vi "Flow_velocity_write.vi"(3 "error in":errorcluster) -> (0 "error out":errorcluster)   [LabVIEW 2013]
uses:
  <vilib>/Analysis/NI_AALPro.lvlib
  <vilib>/Analysis/_algsub.llb/Real Vector Norm.vi
panel:
  in  "NSensors":i32
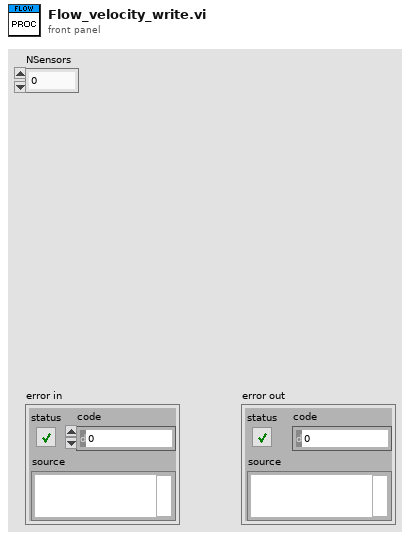
[diagram p1: front panel]
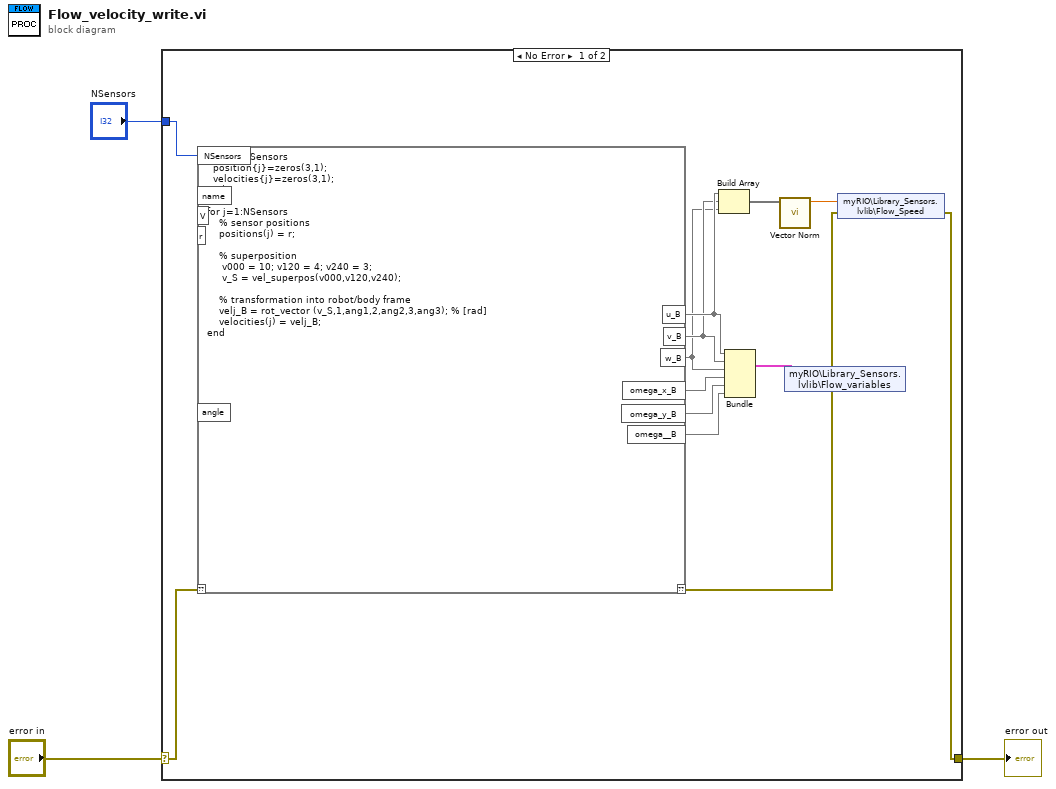
[diagram p0: block diagram]
diagram:
  n1 = case shown="No Error" "error in" {
    selector: "error in" -> [w6 w17]
    tunnel: [w4 w17] -> w2
    tunnel: "NSensors" -> [w12 _]
    frame No Error {
      n2 = mathscript code="for j=1:NSensors\n  position{j}=zeros(3,1);\n  velocities{j}=zeros(3,1);\nend\n\nfor j=1:NSensors\n    % sensor positions\n    positions(j) = r;\n\n    % superposition\n     v000 = 10; v120 = 4; v240 = 3;\n     v_S = vel_superpos(v000,v120,v240);\n\n    % transformation into robot/body frame\n    velj_B = rot_vector (v_S,1,ang1,2,ang2,3,ang3); % [rad]\n    velocities(j) = velj_B;\nend"("??"=w6, "NSensors"=w12) -> ("??"=w5:errorcluster, "u_B"=w11, "v_B"=w10, "w_B"=w9, "omega_x_B"=w15, "omega_y_B"=w14, "omega__B"=w13)  [unwired: 4 in]
      n3 = Build Array(w11, w10, w9) -> (w8:void[])
      n4 = Bundle(w11, w10, w9, w15, w14, w13) -> (w7:cluster{void, void, void, void, void, void})  [unwired: 1 in]
      n5 = call-poly <vilib>:"Vector Norm.vi"("Input Vector"=w8) -> ("norm"=w16:dbl)  [unwired: 9 in, 1 out]
      n6 = shared-variable "myRIO\\Library_Sensors.lvlib\\Flow_variables"(w7) -> ()  [unwired: 1 in, 1 out]
      n7 = shared-variable "myRIO\\Library_Sensors.lvlib\\Flow_Speed"(w16, error in=w5) -> (error out=w4:errorcluster)
    }
    frame Error {
    }
  }
  "error out" <- w2
